vi "Main IU.vi"() -> ()   [LabVIEW 2018]
uses:
  <vilib>/Analysis/baseanly.llb/Mean (DBL).vi
  <vilib>/Utility/file.llb/Read Delimited Spreadsheet (DBL).vi
  <vilib>/Analysis/NI_AALBase.lvlib
panel:
  in  "tiempo 2":dbl
  in  "Setpoint 2":dbl
  in  "Setpoint 1":dbl
  in  "Homing":bool
  out "EsfuerzoSat 2":dbl(graph)
  out "SetpointVsSalida 2":cluster{"Double":dbl, "Output":dbl}(graph)
  out "EsfuerzoSat":dbl(graph)
  out "SetpointVsSalida":cluster{"Double":dbl, "Output":dbl}(graph)
  out "Saving Data":bool
  in  "Record Button":bool
  in  "Filename":path=path "test.lvm"
  out "Motor1":waveform(dbl)[](graph)
  in  "Paro Emergencia:\nUI y RT":bool
  in  "Stop UI":bool
  # "rad"
  # "rad/s"
  # "rad/s^2"
  # "rad/s"
  # "rad/s^2"
  # "s"
  # "rad"
  # "rad"
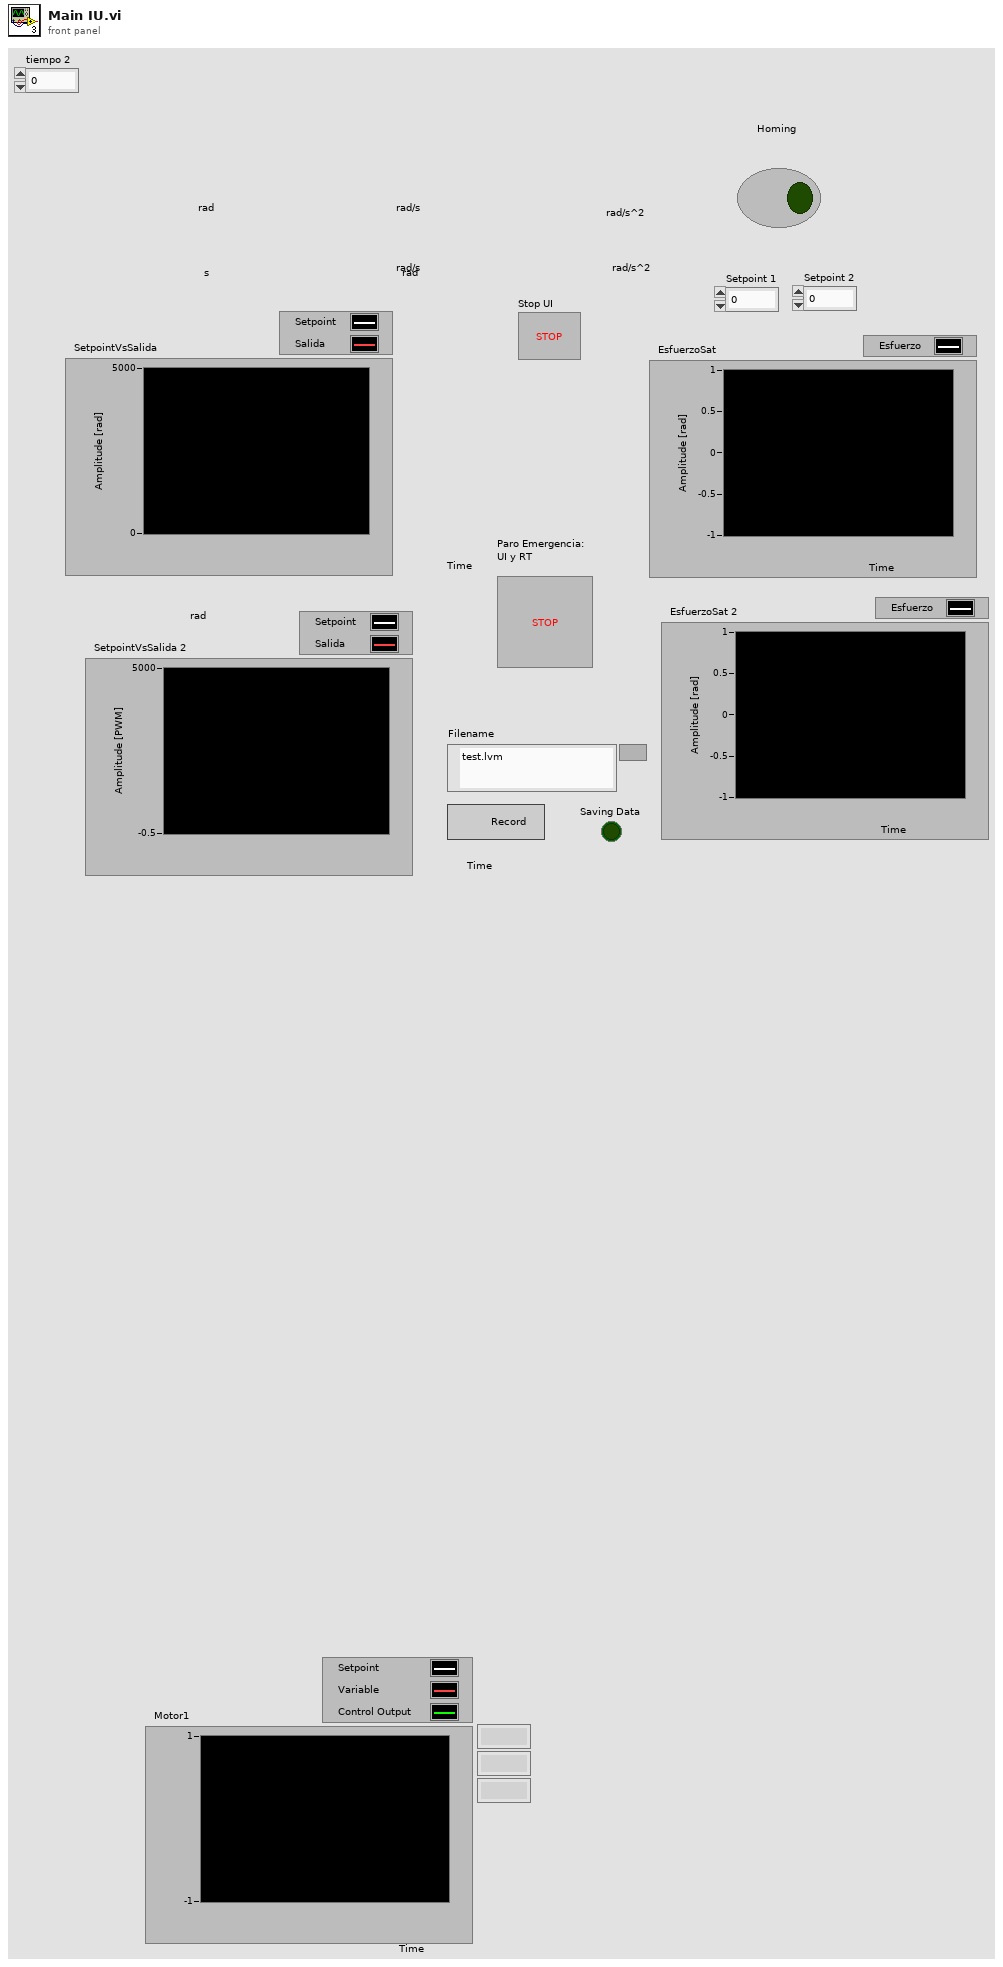
[diagram p1: front panel]
types:
  T1 = cluster{"Double":dbl, "dbl Scaled Value":dbl, "Output":dbl, "seconds since 1Jan1904":timestamp, dbl, dbl, dbl}
  T2 = cluster{"writer name":string, "Variant":variant, "Variant":variant}
  T3 = cluster{"Double":dbl, "dbl Scaled Value":dbl, "Output":dbl, "seconds since 1Jan1904":timestamp, dbl, dbl, dbl}[]
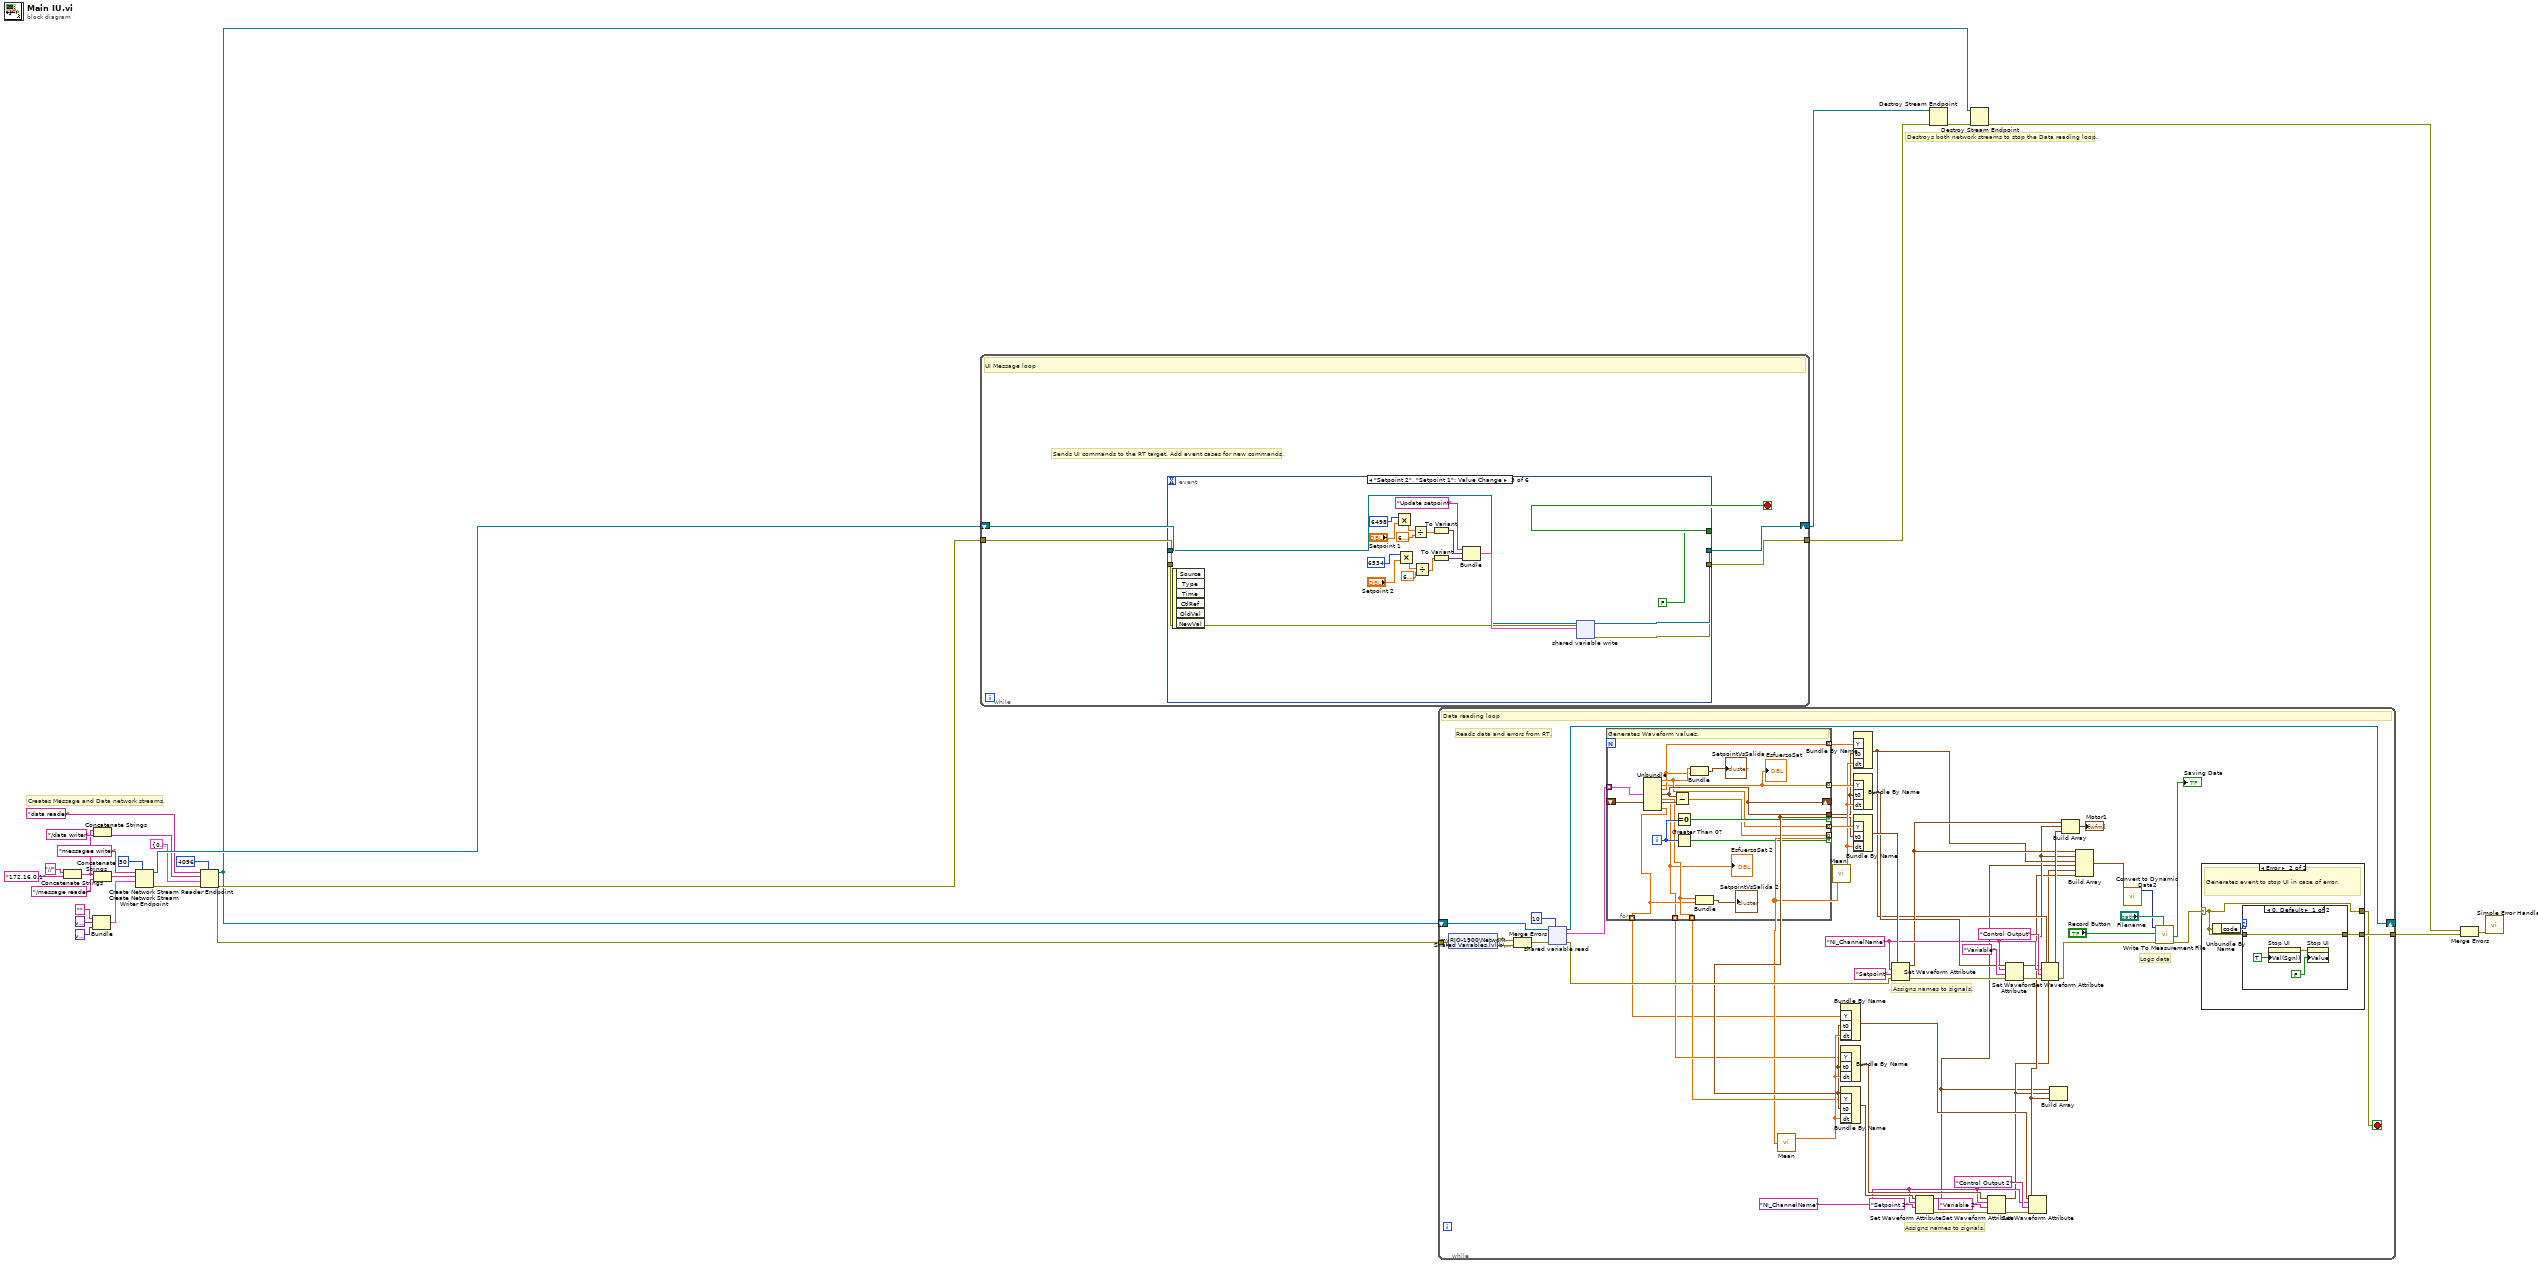
[diagram p0: block diagram]
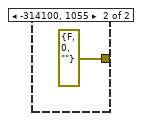
[diagram p3: hidden frame]
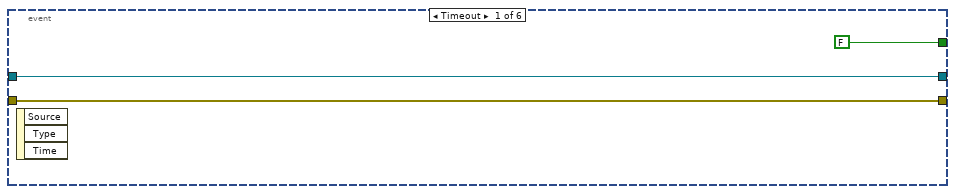
[diagram p4: hidden frame]
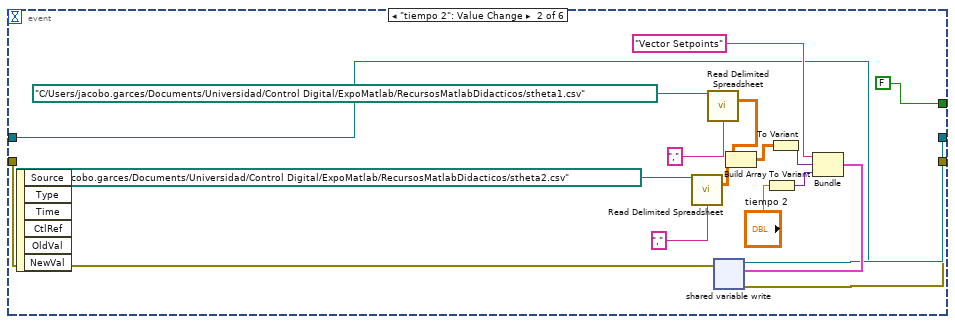
[diagram p5: hidden frame]
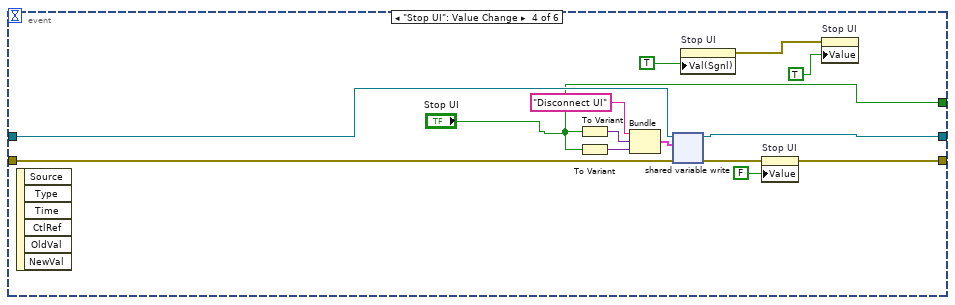
[diagram p6: hidden frame]
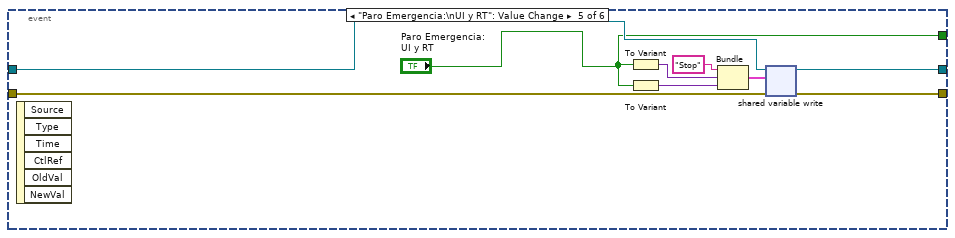
[diagram p7: hidden frame]
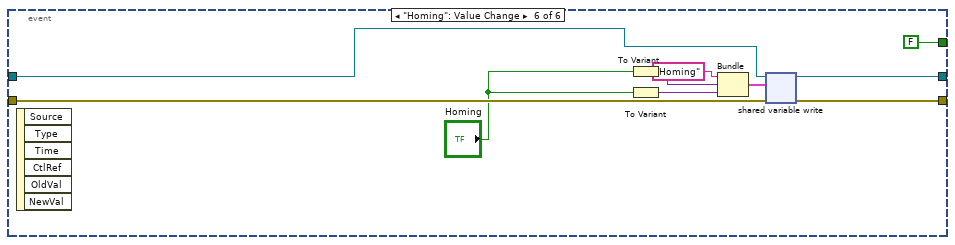
[diagram p8: hidden frame]
diagram:
  # "Destroys both network streams to stop the Data reading loop."
  # "Creates Message and Data network streams."
  n1 = Concatenate Strings("//", "172.16.0.1" ("myRIO IP")) -> (w2:string)
  n2 = Bundle("", variant, variant) -> (w26:cluster{string, variant, variant})  [unwired: 1 in]
  n3 = Concatenate Strings(w2, "/data writer") -> (w17:string)
  n4 = Concatenate Strings(w2, "/message reader") -> (w3:string)
  n5 = Create Network Stream Writer Endpoint(7:50 ("writer buffer size"), 9:w26, 10:w3, 11:"messagee writer" ("writer name")) -> (0:w14:errorcluster, 3:w20:refnum<k21>)  [unwired: 3 in]
  n6 = Create Network Stream Reader Endpoint(7:4096 ("reader buffer size"), 8:w14, 9:T1 {"Double"=0.0, "dbl Scaled Value"=0.0, "Output"=0.0, "seconds since 1Jan1904"=timestamp(0 s since 1904-01-01), 0.0, 0.0, 0.0} ("Data"), 10:w17, 11:"data reader" ("reader name")) -> (0:w13:errorcluster, 3:w6:refnum<k21>)  [unwired: 2 in]
  n7 = while {
    tunnel: w13 -> [w27]
    shift-right: [w31] -> w8
    shift-left: w20 -> [w28]
    tunnel: [w30] -> w9
    stop <- w29 stop-if-true
    # "Sends UI commands to the RT target. Add event cases for new commands."
    # "UI Message loop"
    n8 = event shown="[2] \"Setpoint 2\", \"Setpoint 1\": Value Change" {
      selector: _ -> [_ _ _ _ _ _]
      dyn-events: _ -> [_ _ _ _ _ _]
      timeout: _ -> [_ _ _ _ _ _]
      tunnel: [w33 w46 w65 w81 w89 w99] -> w31
      tunnel: [w32 w45 w64 w78 w90 w100] -> w30
      tunnel: [FALSE ("Stop UI and RT") FALSE ("Stop UI and RT") FALSE ("Stop UI and RT") "Stop UI" "Paro Emergencia:\nUI y RT" FALSE] -> w29
      tunnel: w28 -> [w33 w44 w63 w75 w87 w97]
      tunnel: w27 -> [w32 w43 w62 w76 w86 w96]
      event Timeout {
        n9 = event-data() -> ()  [unwired: 1 in, 3 out]
      }
      event "tiempo 2": Value Change {
        n10 = event-data() -> ()  [unwired: 1 in, 6 out]
        n11 = call-poly <vilib>:"Read Delimited Spreadsheet.vi"("file path (dialog if empty)"=path "C:/Users/jacobo.garces/Documents/Universidad/Control Digital/ExpoMatlab/RecursosMatlabDidacticos/stheta2.csv", "delimiter (\\t)"="," ("delimiter (\\t)")) -> ("all rows"=w38:dbl[][])  [unwired: 8 in, 5 out]
        n12 = call-poly <vilib>:"Read Delimited Spreadsheet.vi"("file path (dialog if empty)"=path "C:/Users/jacobo.garces/Documents/Universidad/Control Digital/ExpoMatlab/RecursosMatlabDidacticos/stheta1.csv", "delimiter (\\t)"="," ("delimiter (\\t)")) -> ("all rows"=w37:dbl[][])  [unwired: 8 in, 5 out]
        n13 = Build Array(w37, w38) -> (w36:dbl[][][])
        n14 = To Variant(anything="tiempo 2") -> (Variant=w49:variant)
        n15 = To Variant(anything=w36) -> (Variant=w47:variant)
        n16 = Bundle("writer name"="Vector Setpoints", "Variant"=w47, "Variant"=w49) -> (w48:T2)  [unwired: 1 in]
        n17 = shared-variable-write(w44, w43, w48) -> (w46:refnum<k21>, w45:errorcluster)  [unwired: 1 in, 1 out]
      }
      event "Setpoint 2", "Setpoint 1": Value Change {
        n18 = event-data() -> ()  [unwired: 1 in, 6 out]
        n19 = Multiply(x=6498, y="Setpoint 1") -> (x*y=w60:dbl)
        n20 = Multiply(x=6534, y="Setpoint 2") -> (x*y=w59:dbl)
        n21 = Divide(x=w60, y=6.283185307179586) -> (x/y=w61:dbl)
        n22 = Divide(x=w59, y=6.283185307179586) -> (x/y=w58:dbl)
        n23 = To Variant(anything=w61) -> (Variant=w66:variant)
        n24 = To Variant(anything=w58) -> (Variant=w68:variant)
        n25 = Bundle("writer name"="Update setpoint", "Variant"=w66, "Variant"=w68) -> (w67:T2)  [unwired: 1 in]
        n26 = shared-variable-write(w63, w62, w67) -> (w65:refnum<k21>, w64:errorcluster)  [unwired: 1 in, 1 out]
      }
      event "Stop UI": Value Change {
        n27 = event-data() -> ()  [unwired: 1 in, 6 out]
        n28 = To Variant(anything="Stop UI") -> (Variant=w84:variant)
        n29 = To Variant(anything="Stop UI") -> (Variant=w77:variant)
        n30 = Bundle("writer name"="Disconnect UI", "Variant"=w84, "Variant"=w77) -> (w83:T2)  [unwired: 1 in]
        n31 = shared-variable-write(w75, w76, w83) -> (w81:refnum<k21>, w79:errorcluster)  [unwired: 1 in, 1 out]
        n32 = property on="Stop UI" class="Bool (strict)"("Val(Sgnl)"=TRUE ("Stop UI and RT")) -> (error out=w74:errorcluster)  [unwired: 2 in, 1 out]
        n33 = property on="Stop UI" class="Bool (strict)"(error in=w79, "Value"=FALSE ("Stop UI and RT")) -> (error out=w78:errorcluster)  [unwired: 1 in, 1 out]
        n34 = property on="Stop UI" class="Bool (strict)"(error in=w74, "Value"=TRUE ("Stop UI")) -> ()  [unwired: 1 in, 2 out]
      }
      event "Paro Emergencia:\nUI y RT": Value Change {
        n35 = event-data() -> ()  [unwired: 1 in, 6 out]
        n36 = To Variant(anything="Paro Emergencia:\nUI y RT") -> (Variant=w93:variant)
        n37 = To Variant(anything="Paro Emergencia:\nUI y RT") -> (Variant=w88:variant)
        n38 = Bundle("writer name"="Stop", "Variant"=w93, "Variant"=w88) -> (w92:T2)  [unwired: 1 in]
        n39 = shared-variable-write(w87, w86, w92) -> (w89:refnum<k21>, w90:errorcluster)  [unwired: 1 in, 1 out]
      }
      event "Homing": Value Change {
        n40 = event-data() -> ()  [unwired: 1 in, 6 out]
        n41 = To Variant(anything="Homing") -> (Variant=w103:variant)
        n42 = To Variant(anything="Homing") -> (Variant=w98:variant)
        n43 = Bundle("writer name"="Homing", "Variant"=w103, "Variant"=w98) -> (w102:T2)  [unwired: 1 in]
        n44 = shared-variable-write(w97, w96, w102) -> (w99:refnum<k21>, w100:errorcluster)  [unwired: 1 in, 1 out]
      }
    }
  }
  n45 = while {
    tunnel: w13 -> [w131]
    shift-right: [w141] -> _
    shift-left: w6 -> [w156]
    tunnel: [w130] -> w10
    stop <- w129 stop-if-true
    w118 = "NI_ChannelName" ("name")
    w135 = "NI_ChannelName" ("name")
    # "Assigns names to signals."
    # "Logs data"
    # "Assigns names to signals."
    # "Reads data and errors from RT."
    # "Data reading loop"
    n46 = shared-variable "myRIO-1900\\Network Shared Variables.lvlib\\error IO"(error in=w131) -> (w134:errorcluster, error out=w133:errorcluster)
    n47 = Merge Errors(w134, w133) -> (w132:errorcluster)
    n48 = shared-variable-read(w156, w132, 10 ("# elements")) -> (w141:refnum<k21>, w146:errorcluster, w154:T3)  [unwired: 1 in, 1 out]
    n49 = for {
      tunnel: w154 -> [w180] mode=indexing
      tunnel: [w173] -> w153 mode=indexing
      tunnel: [w170] -> w152 mode=indexing
      tunnel: [w172] -> w128 mode=indexing
      tunnel: [w178] -> w117 if=w179
      shift-right: [w178] -> _
      shift-left: _ -> [w177]
      tunnel: [w176] -> w114 mode=indexing if=w174
      tunnel: [w167] -> w113 mode=indexing
      tunnel: [w166] -> w116 mode=indexing
      tunnel: [w168] -> w115 mode=indexing
      i -> [w175]
      # "Generates Waveform values."
      n50 = Unbundle(w180) -> ("Double"=w173:dbl, "dbl Scaled Value"=w170:dbl, "Output"=w172:dbl, "seconds since 1Jan1904"=w178:timestamp, w168:dbl, w166:dbl, w167:dbl)
      "EsfuerzoSat" <- w170
      "EsfuerzoSat 2" <- w166
      n51 = Subtract(x=w178, y=w177) -> (x-y=w176:dbl)
      n52 = Equal To 0?(x=w175) -> (x = 0?=w179:bool)
      n53 = Greater Than 0?(x=w175) -> (x > 0?=w174:bool)
      n54 = Bundle("Double"=w173, "Output"=w172) -> (→"SetpointVsSalida":cluster{"Double":dbl, "Output":dbl})  [unwired: 1 in]
      n55 = Bundle(w168, w167) -> (→"SetpointVsSalida 2":cluster{dbl, dbl})  [unwired: 1 in]
    }
    n56 = call-poly <vilib>:"Mean.vi"("X"=w114) -> ("mean"=w127:dbl)  [unwired: 1 out]
    n57 = call-poly <vilib>:"Mean.vi"("X"=w114) -> ("mean"=w151:dbl)  [unwired: 1 out]
    n58 = Bundle By Name("Y"=w113, "t0"=w117, "dt"=w127) -> (w119:waveform(dbl))  [unwired: 1 in]
    n59 = Bundle By Name("Y"=w116, "t0"=w117, "dt"=w127) -> (w120:waveform(dbl))  [unwired: 1 in]
    n60 = Bundle By Name("Y"=w115, "t0"=w117, "dt"=w127) -> (w126:waveform(dbl))  [unwired: 1 in]
    n61 = Bundle By Name("Y"=w128, "t0"=w117, "dt"=w151) -> (w109:waveform(dbl))  [unwired: 1 in]
    n62 = Bundle By Name("Y"=w152, "t0"=w117, "dt"=w151) -> (w143:waveform(dbl))  [unwired: 1 in]
    n63 = Bundle By Name("Y"=w153, "t0"=w117, "dt"=w151) -> (w150:waveform(dbl))  [unwired: 1 in]
    n64 = Set Waveform Attribute(4:w146, 5:"Setpoint" ("name"), 6:w135, 7:w150) -> (0:w145:errorcluster, 3:w110:waveform(dbl))  [unwired: 1 out]
    n65 = Set Waveform Attribute(5:"Setpoint 2" ("name"), 6:w118, 7:w126) -> (0:w122:errorcluster, 3:w105:waveform(dbl))  [unwired: 1 in, 1 out]
    n66 = Set Waveform Attribute(4:w122, 5:"Variable 2" ("name"), 6:w118, 7:w120) -> (0:w121:errorcluster, 3:w106:waveform(dbl))  [unwired: 1 out]
    n67 = Set Waveform Attribute(4:w145, 5:"Variable" ("name"), 6:w135, 7:w143) -> (0:w144:errorcluster, 3:w108:waveform(dbl))  [unwired: 1 out]
    n68 = Set Waveform Attribute(4:w121, 5:"Control Output 2" ("name"), 6:w118, 7:w119) -> (3:w107:waveform(dbl))  [unwired: 2 out]
    n69 = Set Waveform Attribute(4:w144, 5:"Control Output" ("name"), 6:w135, 7:w109) -> (0:w140:errorcluster, 3:w142:waveform(dbl))  [unwired: 1 out]
    n70 = Build Array(w105, w106, w107) -> ()  [unwired: 1 out]
    n71 = Build Array(w110, w108, w142) -> (→"Motor1":waveform(dbl)[])
    n72 = Build Array(w110, w108, w109, w105, w106, w107) -> (w104:waveform(dbl)[])
    n73 = call "Convert to Dynamic Data2"("Array of Waveforms"=w104) -> ("Dynamic Data Type"=w111:dynamicdata)  [unwired: 3 in]
    n74 = call "Write To Measurement File"("Signals"=w111, "Enable"="Record Button", "error in (no error)"=w140, "Filename"="Filename") -> ("Saving Data"=→"Saving Data":bool, "error out"=w136:errorcluster)  [unwired: 13 in, 1 out]
    n75 = case shown="Error" w136 {
      selector: w136 -> [w157 w158]
      tunnel: [w157 w159] -> w130
      tunnel: [w157 w158] -> w129
      frame No Error {
        # "No action required."
      }
      frame Error {
        # "Generates event to stop UI in case of error."
        n76 = Unbundle By Name(w158) -> ("code"=w160:i32)
        n77 = case shown="0, Default" w160 {
          tunnel: [w163 errorcluster {"status"=FALSE, "code"=0, "source"=""} ("error IO")] -> w159
          tunnel: w158 -> [w163 _]
          frame 0, Default {
            n78 = property on="Stop UI" class="Bool (strict)"("Val(Sgnl)"=TRUE ("Stop UI and RT")) -> (error out=w162:errorcluster)  [unwired: 2 in, 1 out]
            n79 = property on="Stop UI" class="Bool (strict)"(error in=w162, "Value"=FALSE ("Stop UI")) -> ()  [unwired: 1 in, 2 out]
          }
          frame -314100, 1055 {
          }
        }
      }
    }
  }
  n80 = Destroy Stream Endpoint(8:w9, 11:w8) -> (0:w7:errorcluster)
  n81 = Destroy Stream Endpoint(8:w7, 11:w6) -> (0:w5:errorcluster)
  n82 = Merge Errors(w5, w10) -> (w11:errorcluster)
  n83 = call <vilib>:"Simple Error Handler.vi"("error in (no error)"=w11) -> ()  [unwired: 4 in, 5 out]
